vi "Stepper StoppedEvent Example.vi"() -> ()   [LabVIEW 2012, in "Phidget Stepper.lvlib"]
uses:
  <instrlib>/Phidgets/Phidget Stepper/Phidget Stepper.lvlib
  <instrlib>/Phidgets/Phidget Stepper/Public/StepperStart.vi
  <instrlib>/Phidgets/Phidget Stepper/Public/StepperClose.vi
  <instrlib>/Phidgets/Phidget Common/Phidget Common.lvlib
panel:
  in  "Stepper Initialization Data":T1={"Control Mode"=0, " Rescale Factor"=1.0, "Velocity Limit"=10000.0, "Acceleration"=10000.0, "Current Limit"=1.0} {"Control Mode" items=["Step", "Run"]}
  in  "Target Position Position":dbl
  out "Event?":bool
  in  "stop":bool
  out "Serial Number Return":i32
  in  "Device Info":T2={"Serial Number"=-1, "Channel"=0, "Port"=0}
  out "error out":errorcluster
  # "Be sure to use this stop button to stop the program.\nIf you use the \"Abort Execution\" button, you will\nneed to use PhidgetResetLibrary.vi or restart Labview \nin order for any Phidgets to work."
  # "NOTE: The default\nVelocity Limit and\nAcceleration\nparameters will not\nwork with the 1062.\nThese may be\nboth set to 200\n(or any other value \nin the valid range)\nfor the device to\nwork."
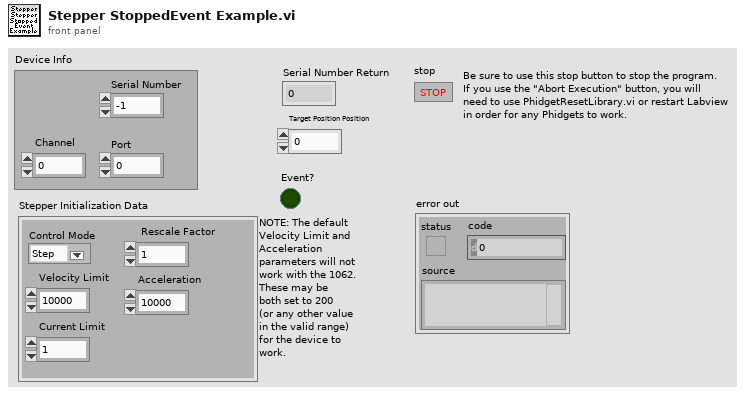
[diagram p1: front panel]
types:
  T1 = cluster{"Control Mode":u16, " Rescale Factor":dbl, "Velocity Limit":dbl, "Acceleration":dbl, "Current Limit":dbl}
  T2 = cluster{"Serial Number":i32, "Channel":i32, "Port":i32}
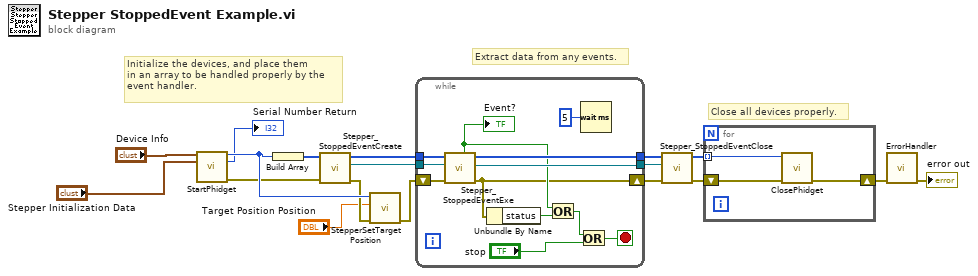
[diagram p0: block diagram]
diagram:
  # "Close all devices properly."
  # "Extract data from any events."
  # "Initialize the devices, and place them\nin an array to be handled properly by the\nevent handler."
  n1 = call-poly <instrlib>:"StartPhidget.vi"("Device Info"="Device Info", "Stepper Initialization Data"="Stepper Initialization Data") -> ("Phidget ID"=w7:u64, "Serial Number Return"=→"Serial Number Return":i32, "error out"=w1:errorcluster)  [unwired: 10 in, 1 out]
  n2 = Build Array(w7) -> (w18:u64[])
  n3 = call <instrlib>:"Stepper_StoppedEventCreate.vi"("error in (no error)"=w1, "Devices In"=w18) -> ("error out"=w6:errorcluster, "Event Registration Refnum"=w16:refnum<event-registration>, "Devices Out"=w17:u64[])  [unwired: 7 in]
  n4 = call <instrlib>:"StepperSetTargetPosition.vi"("error in (no error)"=w6, "Target Position Position"="Target Position Position", "Device In"=w7) -> ("error out"=w5:errorcluster)  [unwired: 6 in, 1 out]
  n5 = while {
    tunnel: w17 -> [w30]
    tunnel: w16 -> [w25]
    tunnel: [w29] -> w13
    shift-right: [w19] -> w12
    shift-left: w5 -> [w28]
    tunnel: [w26] -> w8
    stop <- w24 stop-if-true
    n6 = call <instrlib>:"Stepper_StoppedEventExe.vi"("error in (no error)"=w28, "Event Registration Refnum In"=w25, "Devices In"=w30) -> ("error out"=w19:errorcluster, "Event Registration Refnum Out"=w29:refnum<event-registration>, "Devices Out"=w26:u64[], "Event?"=w20:bool)  [unwired: 3 in, 2 out]
    "Event?" <- w20
    n7 = Unbundle By Name(w19) -> ("status"=w21:bool)
    n8 = Or(x=w20, y=w21) -> (x .or. y?=w22:bool)
    n9 = Or(x=w22, y="stop") -> (x .or. y?=w24:bool)
    n10 = Wait (ms)(milliseconds to wait=u32 5) -> ()  [unwired: 1 out]
  }
  n11 = call <instrlib>:"Stepper_StoppedEventClose.vi"("error in (no error)"=w12, "Event Registration Refnum In"=w13, "Devices In"=w8) -> ("error out"=w10:errorcluster, "Devices Out"=w9:u64[])  [unwired: 7 in]
  n12 = for {
    tunnel: w9 -> [w31] mode=indexing
    shift-right: [w33] -> w15
    shift-left: w10 -> [w32]
    n13 = call-poly <instrlib>:"ClosePhidget.vi"("error in"=w32, "Device In"=w31) -> ("error out"=w33:errorcluster)  [unwired: 9 in]
  }
  n14 = call <instrlib>:"ErrorHandler.vi"("error in"=w15) -> ("error out"=→"error out":errorcluster)  [unwired: 9 in, 1 out]
